vi "isOpen.vi"(8 "error in (no error)":errorcluster, 11 "Monochromator in":refnum<class "Monochromator.lvclass">) -> (0 "error out":errorcluster, 2 "CCD is open?":T1, 3 "Monochromator out":refnum<class "Monochromator.lvclass">)   [LabVIEW 2023, in "Monochromator.lvclass"]
uses:
  Monochromator.lvclass
  Monochromator.lvclass/Monochromator.ctl
  d9b87029-586e-44ee-a6e5-d4a5e0edce38.vi
  b59fd1e7-dcda-425c-bd6c-61aafb79e7f4.vi
  GenericDevice/GenericDevice.lvclass
  monoIsOpen.ctl
  CCD/IsOpen.ctl
  CCD/CCD.lvclass
panel:
  # "Connector Pane"
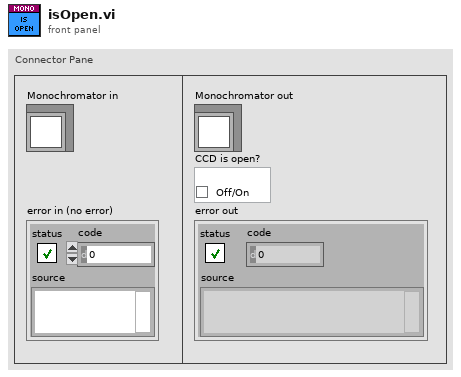
[diagram p1: front panel]
types:
  T1 = typedef "CCD.lvclass/IsOpen.ctl" = cluster{"isOpen":bool}
  T2 = typedef "Monochromator.lvclass/monoIsOpen.ctl" = cluster{"Checkbox":bool}
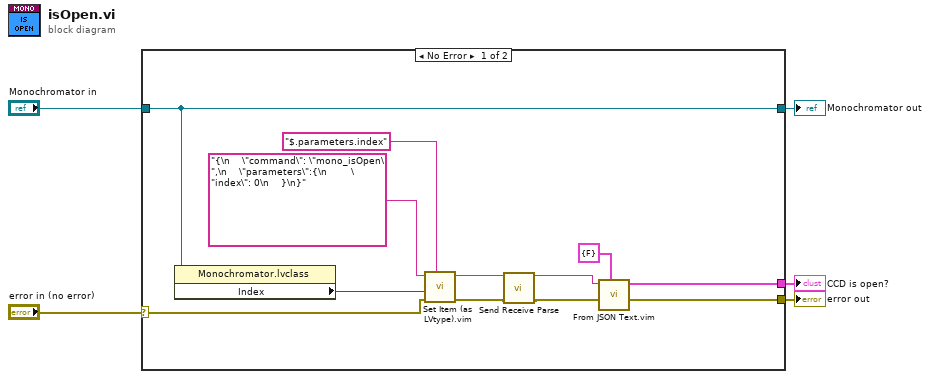
[diagram p0: block diagram]
diagram:
  n1 = case shown="No Error" "error in (no error)" {
    selector: "error in (no error)" -> [w13 w19]
    tunnel: [w11 w19] -> w4
    tunnel: [w15 w18] -> w1
    tunnel: "Monochromator in" -> [w15 w18]
    tunnel: [w12 _] -> w3
    frame No Error {
      n2 = property class="Monochromator.lvclass"(reference=w15) -> ("Index"=w14:i32)  [unwired: 1 in, 2 out]
      n3 = call "Set Item (as LVtype).vim"("$Path or Item Name"="$.parameters.index", "error in (no error)"=w13, "Anything"=w14, "JSON"="{\n    \"command\": \"mono_isOpen\",\n    \"parameters\":{\n        \"index\": 0\n    }\n}") -> ("error out"=w9:errorcluster, "<JSON>"=w10:string)  [unwired: 4 in, 1 out]
      n4 = call "Send Receive Parse.vi"("<JSON>"=w10, "error in"=w9) -> ("results-JSON string"=w8:string, "error out"=w7:errorcluster)  [unwired: 9 in, 3 out]
      n5 = call "From JSON Text.vim"("Data Type and Default Value"=T2 {"Checkbox"=FALSE} ("Cluster"), "error in (no error)"=w7, "JSON"=w8) -> ("error out"=w11:errorcluster, "Data out"=w12:T2)  [unwired: 7 in]
    }
    frame Error {
    }
  }
  "error out" <- w4
  "CCD is open?" <- w3
  "Monochromator out" <- w1
